vi "External Actuator Settings DAO.vi"(7 "refnum":T2, 8 "error in (no error)":errorcluster, 9 "External Actuator Id":T1, 10 "Actuator Settings In":T3, 11 "Persistent DAO Actions":T5) -> (0 "error out":errorcluster, 2 "Actuator Settings Out":T3, 4 "refnum out":T2)   [LabVIEW 2009]
uses:
  Metadata/Persistant DAO Actions.ctl
  External Actuator Settings.ctl
  Apps/Yes No Button.ctl
  <vilib>/Utility/config.llb/Config Data RefNum.ctl
  External Actuator Id.ctl
  <vilib>/Utility/config.llb/Read Key (Boolean).vi
  <vilib>/Utility/config.llb/Read Key (Double).vi
  <vilib>/Utility/config.llb/Write Key (Boolean).vi
  <vilib>/Utility/config.llb/Write Key (Double).vi
  <vilib>/Utility/config.llb/NI_LVConfig.lvlib
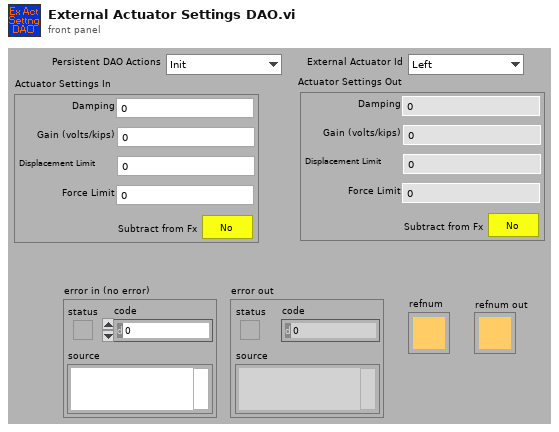
[diagram p1: front panel]
types:
  T1 = typedef "External Actuator Id.ctl" = enum16{"Left", "Right"}
  T2 = typedef "NI_LVConfig.lvlib/Config Data RefNum.ctl" = refnum<k1>
  T3 = typedef "External Actuator Settings.ctl" = cluster{"Displacement Limit":dbl, "Damping":dbl, "Gain (volts/kips)":dbl, "Subtract from Fx":T4, "Force Limit":dbl}
  T4 = typedef "Yes No Button.ctl" = bool
  T5 = typedef "Persistant DAO Actions.ctl" = enum16{"Init", "Get", "Set", "Load", "Save"}
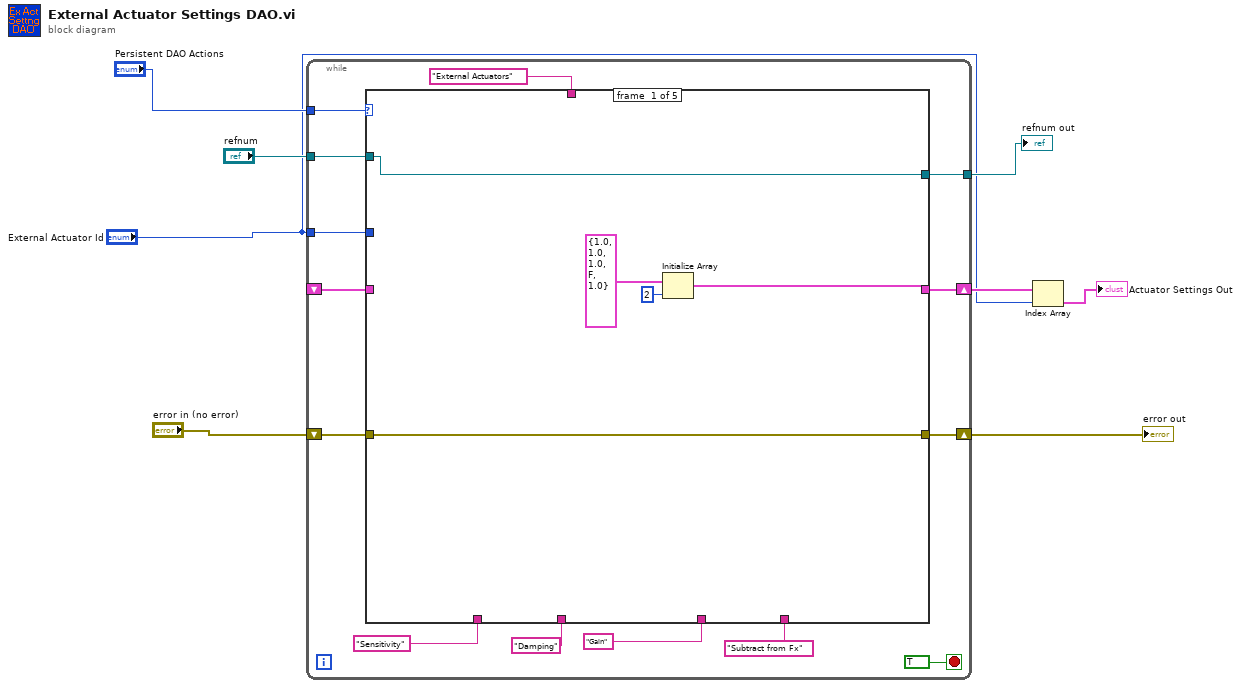
[diagram p0: block diagram]
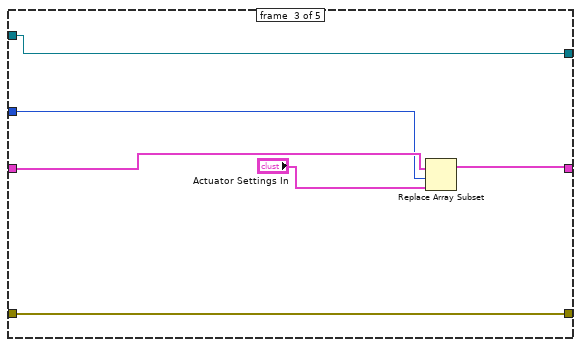
[diagram p3: hidden frame]
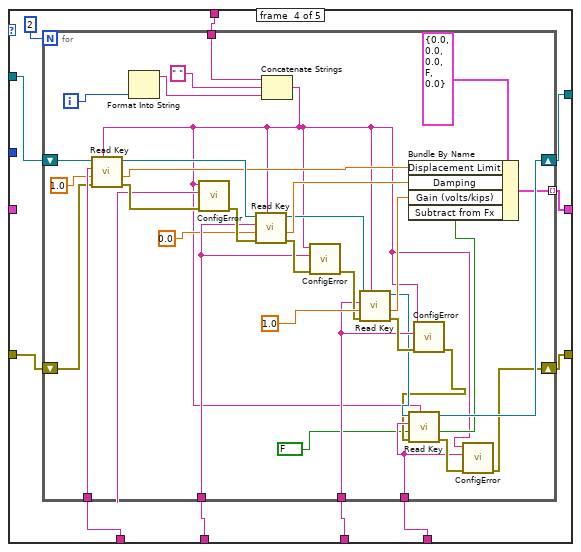
[diagram p4: hidden frame]
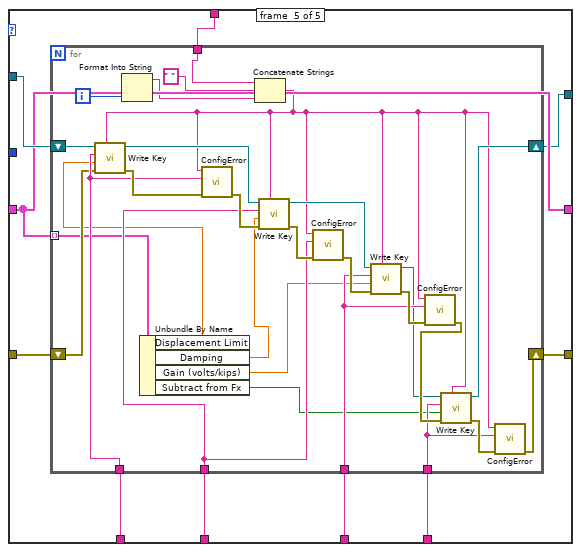
[diagram p5: hidden frame]
diagram:
  n1 = while {
    tunnel: "Persistent DAO Actions" -> [w21]
    shift-right: [w12] -> w7
    shift-left: _ -> [w13]
    tunnel: "refnum" -> [w18]
    shift-right: [w15] -> w4
    shift-left: "error in (no error)" -> [w16]
    tunnel: [w14] -> w3
    tunnel: "External Actuator Id" -> [w9]
    stop <- TRUE stop-if-true
    n2 = case shown="\"Load\"" w21 {
      tunnel: "External Actuators" -> [_ _ _ w39 w81]
      tunnel: "Sensitivity" -> [_ _ _ w47 w90]
      tunnel: w18 -> [w27 w29 w35 w46 w89]
      tunnel: "Damping" -> [_ _ _ w45 w88]
      tunnel: w16 -> [w26 w30 w36 w44 w87]
      tunnel: [w26 w30 w36 w40 w84] -> w15
      tunnel: [w27 w29 w35 w41 w82] -> w14
      tunnel: w13 -> [_ w28 w32 _ w86]
      tunnel: [w24 w28 w34 w38 w86] -> w12
      tunnel: "Gain" -> [_ _ _ w43 w85]
      tunnel: "Subtract from Fx" -> [_ _ _ w42 w83]
      tunnel: w9 -> [_ _ w31 _ _]
      frame #0 {
        n3 = Initialize Array(T3 {"Displacement Limit"=1.0, "Damping"=1.0, "Gain (volts/kips)"=1.0, "Subtract from Fx"=FALSE, "Force Limit"=1.0} ("Autobalance Control In"), 2 ("dimension size")) -> (w24:T3[])
      }
      frame #1 {
      }
      frame #2 {
        n4 = Replace Array Subset(array=w32, new element="Actuator Settings In", index=w31) -> (w34:T3[])
      }
      frame #3 {
        n5 = for {
          N: 2 -> [_]
          tunnel: w47 -> [w79]
          tunnel: w45 -> [w74]
          tunnel: w43 -> [w63]
          tunnel: w42 -> [w60]
          tunnel: w39 -> [w50]
          tunnel: [w54] -> w38 mode=indexing
          shift-right: [w58] -> w41
          shift-left: w46 -> [w78]
          shift-right: [w56] -> w40
          shift-left: w44 -> [w72]
          i -> [w48]
          n6 = Format Into String(w48) -> (resulting string=w52:string)  [unwired: 3 in, 1 out]
          n7 = Concatenate Strings(w50, " " ("string"), w52) -> (w49:string)
          n8 = call-poly <vilib>:"Read Key.vi"("section"=w49, "error in (no error)"=w72, "default value"=1.0 ("Port Number In"), "key"=w79, "refnum"=w78) -> ("error out"=w80:errorcluster, "value"=w69:dbl, "refnum out"=w75:T2)  [unwired: 4 out]
          n9 = call "ConfigError.vi"("error in (no error)"=w80, "Key"=w79, "Section"=w49) -> ("error out"=w76:errorcluster)  [unwired: 8 out]
          n10 = call-poly <vilib>:"Read Key.vi"("section"=w49, "error in (no error)"=w76, "default value"=0.0 ("Wait For Notification Timeout In"), "key"=w74, "refnum"=w75) -> ("error out"=w77:errorcluster, "value"=w68:dbl, "refnum out"=w66:T2)  [unwired: 4 out]
          n11 = call "ConfigError.vi"("error in (no error)"=w77, "Key"=w74, "Section"=w49) -> ("error out"=w64:errorcluster)  [unwired: 8 out]
          n12 = call-poly <vilib>:"Read Key.vi"("section"=w49, "error in (no error)"=w64, "default value"=1.0, "key"=w63, "refnum"=w66) -> ("error out"=w67:errorcluster, "value"=w62:dbl, "refnum out"=w59:T2)  [unwired: 4 out]
          n13 = call "ConfigError.vi"("error in (no error)"=w67, "Key"=w63, "Section"=w49) -> ("error out"=w57:errorcluster)  [unwired: 8 out]
          n14 = call-poly <vilib>:"Read Key.vi"("section"=w49, "error in (no error)"=w57, "default value"=FALSE, "key"=w60, "refnum"=w59) -> ("error out"=w61:errorcluster, "value"=w55:bool, "refnum out"=w58:T2)  [unwired: 4 out]
          n15 = Bundle By Name(cluster=T3 {"Displacement Limit"=0.0, "Damping"=0.0, "Gain (volts/kips)"=0.0, "Subtract from Fx"=FALSE, "Force Limit"=0.0} ("Autobalance Control In"), "Displacement Limit"=w69, "Damping"=w68, "Gain (volts/kips)"=w62, "Subtract from Fx"=w55) -> (w54:T3)
          n16 = call "ConfigError.vi"("error in (no error)"=w61, "Key"=w60, "Section"=w49) -> ("error out"=w56:errorcluster)  [unwired: 8 out]
        }
      }
      frame #4 {
        n17 = for {
          tunnel: w90 -> [w117]
          tunnel: w88 -> [w112]
          tunnel: w86 -> [w110] mode=indexing
          tunnel: w85 -> [w104]
          tunnel: w83 -> [w99]
          tunnel: w81 -> [w93]
          shift-right: [w96] -> w82
          shift-left: w89 -> [w116]
          shift-right: [w100] -> w84
          shift-left: w87 -> [w111]
          i -> [w91]
          n18 = Format Into String(w91) -> (resulting string=w95:string)  [unwired: 3 in, 1 out]
          n19 = Unbundle By Name(w110) -> ("Displacement Limit"=w109:dbl, "Damping"=w108:dbl, "Gain (volts/kips)"=w103:dbl, "Subtract from Fx"=w98:T4)
          n20 = Concatenate Strings(w93, " " ("string"), w95) -> (w92:string)
          n21 = call-poly <vilib>:"Write Key.vi"("section"=w92, "error in (no error)"=w111, "value"=w109, "key"=w117, "refnum"=w116) -> ("error out"=w118:errorcluster, "refnum out"=w113:T2)  [unwired: 3 in, 2 out]
          n22 = call "ConfigError.vi"("error in (no error)"=w118, "Key"=w117, "Section"=w92) -> ("error out"=w114:errorcluster)  [unwired: 8 out]
          n23 = call-poly <vilib>:"Write Key.vi"("section"=w92, "error in (no error)"=w114, "value"=w108, "key"=w112, "refnum"=w113) -> ("error out"=w115:errorcluster, "refnum out"=w105:T2)  [unwired: 3 in, 2 out]
          n24 = call "ConfigError.vi"("error in (no error)"=w115, "Key"=w112, "Section"=w92) -> ("error out"=w106:errorcluster)  [unwired: 8 out]
          n25 = call-poly <vilib>:"Write Key.vi"("section"=w92, "error in (no error)"=w106, "value"=w103, "key"=w104, "refnum"=w105) -> ("error out"=w107:errorcluster, "refnum out"=w97:T2)  [unwired: 3 in, 2 out]
          n26 = call "ConfigError.vi"("error in (no error)"=w107, "Key"=w104, "Section"=w92) -> ("error out"=w101:errorcluster)  [unwired: 8 out]
          n27 = call-poly <vilib>:"Write Key.vi"("section"=w92, "error in (no error)"=w101, "value"=w98, "key"=w99, "refnum"=w97) -> ("error out"=w102:errorcluster, "refnum out"=w96:T2)  [unwired: 5 out]
          n28 = call "ConfigError.vi"("error in (no error)"=w102, "Key"=w99, "Section"=w92) -> ("error out"=w100:errorcluster)  [unwired: 8 out]
        }
      }
    }
  }
  "error out" <- w4
  "refnum out" <- w3
  n29 = Index Array(array=w7, index="External Actuator Id") -> (element=→"Actuator Settings Out":T3)
